vi "Demo - Read 1 Analog Sample on Demand.vi"() -> ()   [LabVIEW 2020]
panel:
  out "Waveform Chart":dbl(graph)
  in  "stop":bool
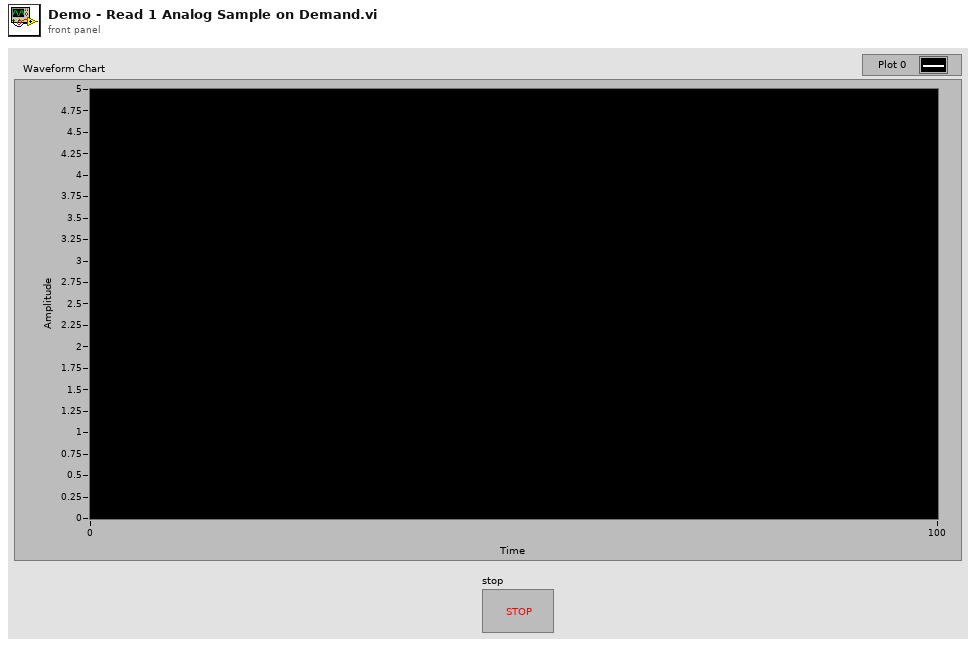
[diagram p1: front panel]
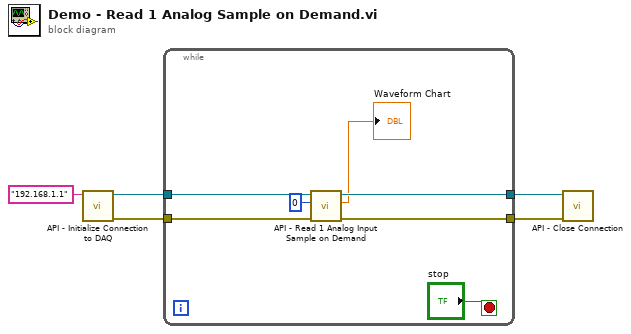
[diagram p0: block diagram]
diagram:
  n1 = call "API - Initialize Connection to DAQ.vi"("DAQ IP Address"="192.168.1.1") -> ("error out"=w2:errorcluster, "TCP Network Connection out"=w5:refnum<k5>)  [unwired: 9 in]
  n2 = while {
    tunnel: w5 -> [w11]
    tunnel: [w10] -> w4
    tunnel: [w9] -> w3
    tunnel: w2 -> [w8]
    stop <- "stop" stop-if-true
    n3 = call "API - Read 1 Analog Input Sample on Demand.vi"("error in"=w8, "Analog Input Channel Number"=0, "TCP Network Connection in"=w11) -> ("error out"=w9:errorcluster, "Data Out"=→"Waveform Chart":dbl, "TCP Network Connection out"=w10:refnum<k5>)  [unwired: 6 in]
  }
  n4 = call "API - Close Connection.vi"("error in"=w3, "TCP Network Connection in"=w4) -> ()  [unwired: 9 in, 1 out]
